vi "Download Record.vi"(0 "Instrument Handle In":i32, 1 "Start Time":dbl format="%^#_6g", 5 "Source":i32(ring) items=["Input Channel 1", "Input Channel 2", "Input Channel 3", "Input Channel 4", "Calc Channel 1", "Calc Channel 2", "Calc Channel 3", "Calc Channel 4", "Ref Channel 1", "Ref Channel 2", "Ref Channel 3", "Ref Channel 4"], 7 "Points":i32=1000, 9 "Transfer Type":i32(ring)=2 items=["s8", "s16", "s32", "f32", "f64"], 11 "error in":errorcluster, 12 "Stop Time":dbl format="%^#_6g") -> (3 "F64 Wave":dbl[](array[numeric]), 4 "Instrument Handle Out":i32, 6 "S8 Wave":i8[](array[numeric]), 8 "S16 Wave":i16[](array[numeric]), 10 "S32 Wave":i32[](array[numeric]), 14 "F32 Wave":sgl[](array[numeric]), 15 "error out":errorcluster)   [LabVIEW 2013, in "ZTScopeM.lvlib"]
doc: "Read the waveform in the source channel. The returned data format depends on the Transfer Type. Use \"Read Waveform Preamble\" to get the appropriate time and magnitude bases."
uses:
  ZTScopeM.lvlib
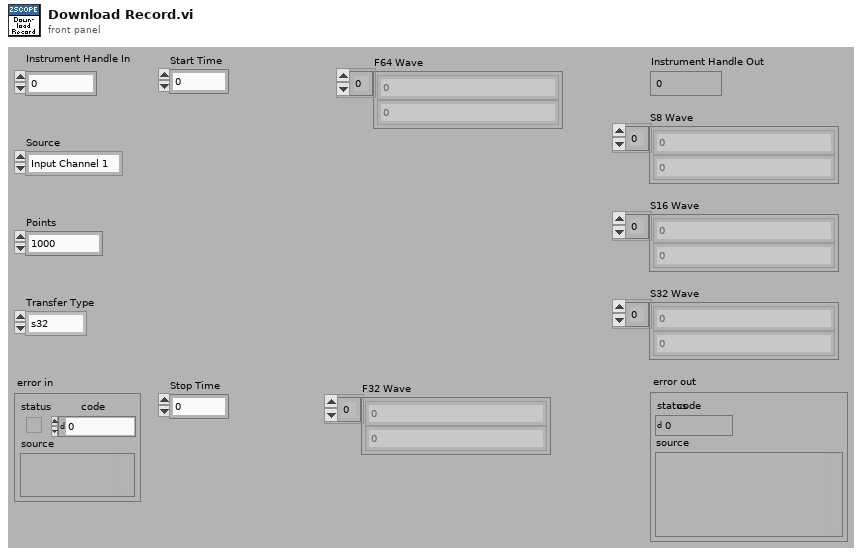
[diagram p1: front panel]
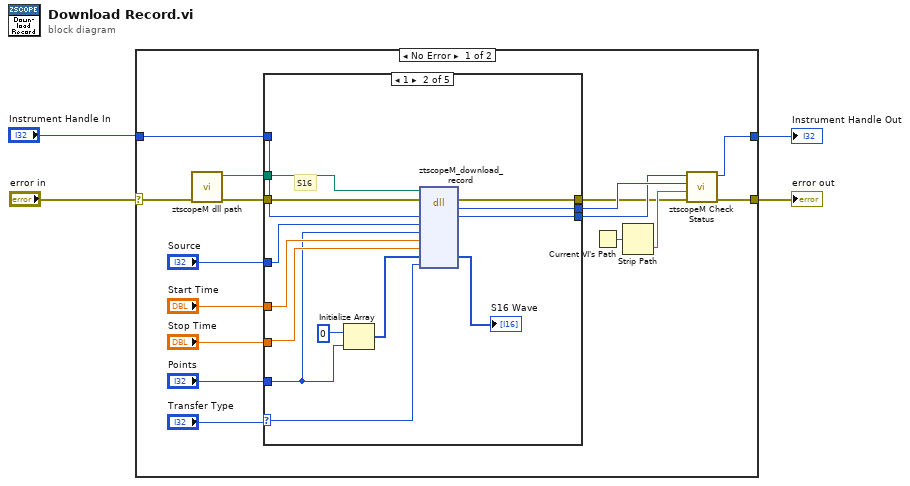
[diagram p0: block diagram]
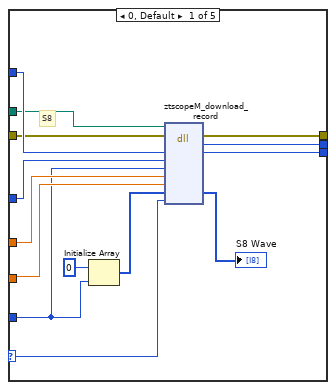
[diagram p2: hidden frame]
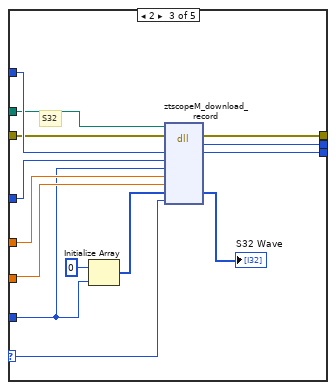
[diagram p3: hidden frame]
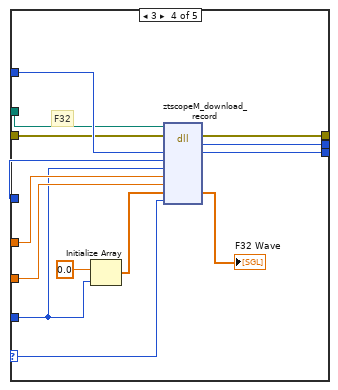
[diagram p4: hidden frame]
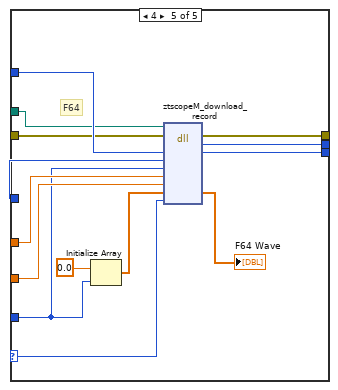
[diagram p5: hidden frame]
diagram:
  n1 = case shown="No Error" "error in" {
    selector: "error in" -> [w8 w92]
    tunnel: [w15 w92] -> w1
    tunnel: "Instrument Handle In" -> [w14 w91]
    tunnel: [w16 w91] -> w3
    frame No Error {
      n2 = call "ztscopeM dll path.vi"("error in (no error)"=w8) -> ("error out"=w6:errorcluster, "<instrument>.dll path"=w7:path)  [unwired: 9 in]
      n3 = case shown="1" "Transfer Type" {
        selector: "Transfer Type" -> [w25 w39 w53 w67 w81]
        tunnel: [w27 w41 w55 w75 w89] -> w18
        tunnel: [w26 w40 w54 w74 w88] -> w17
        tunnel: w14 -> [w28 w42 w56 w73 w87]
        tunnel: "Points" -> [w24 w38 w52 w66 w80]
        tunnel: "Source" -> [w29 w43 w57 w72 w86]
        tunnel: "Start Time" -> [w30 w44 w58 w69 w83]
        tunnel: "Stop Time" -> [w31 w45 w59 w68 w82]
        tunnel: w7 -> [w23 w37 w51 w65 w79]
        tunnel: w6 -> [w22 w36 w49 w64 w78]
        tunnel: [w21 w35 w50 w63 w77] -> w5
        frame 0, Default {
          # "S8"
          n4 = Initialize Array(i8 0, w24) -> (w33:i8[])
          n5 = dll-call lib="C:/Program Files (x86)/National Instruments/LabVIEW 2013/instr.lib/ztscopem/ztscopeM.dll" fn="ztscopeM_download_record"(path in=w23, error in=w22, "instrumentHandle"=w28, "source"=w29, "points"=w24, "startTime"=w30, "stopTime"=w31, "Waveform"=w33, "transferType"=w25) -> (error out=w21:errorcluster, w27:i32, "instrumentHandle"=w26:i32, "Waveform"=→"S8 Wave":i8[])  [unwired: 6 in, 1 out]
        }
        frame 1 {
          # "S16"
          n6 = Initialize Array(i16 0, w38) -> (w47:i16[])
          n7 = dll-call lib="C:/Program Files (x86)/National Instruments/LabVIEW 2013/instr.lib/ztscopem/ztscopeM.dll" fn="ztscopeM_download_record"(path in=w37, error in=w36, "instrumentHandle"=w42, "source"=w43, "points"=w38, "startTime"=w44, "stopTime"=w45, "Waveform"=w47, "transferType"=w39) -> (error out=w35:errorcluster, w41:i32, "instrumentHandle"=w40:i32, "Waveform"=→"S16 Wave":i16[])  [unwired: 6 in, 1 out]
        }
        frame 2 {
          # "S32"
          n8 = Initialize Array(0, w52) -> (w61:i32[])
          n9 = dll-call lib="C:/Program Files (x86)/National Instruments/LabVIEW 2013/instr.lib/ztscopem/ztscopeM.dll" fn="ztscopeM_download_record"(path in=w51, error in=w49, "instrumentHandle"=w56, "source"=w57, "points"=w52, "startTime"=w58, "stopTime"=w59, "Waveform"=w61, "transferType"=w53) -> (error out=w50:errorcluster, w55:i32, "instrumentHandle"=w54:i32, "Waveform"=→"S32 Wave":i32[])  [unwired: 6 in, 1 out]
        }
        frame 3 {
          # "F32"
          n10 = Initialize Array(sgl 0.0, w66) -> (w71:sgl[])
          n11 = dll-call lib="C:/Program Files (x86)/National Instruments/LabVIEW 2013/instr.lib/ztscopem/ztscopeM.dll" fn="ztscopeM_download_record"(path in=w65, error in=w64, "instrumentHandle"=w73, "source"=w72, "points"=w66, "startTime"=w69, "stopTime"=w68, "Waveform"=w71, "transferType"=w67) -> (error out=w63:errorcluster, w75:i32, "instrumentHandle"=w74:i32, "Waveform"=→"F32 Wave":sgl[])  [unwired: 6 in, 1 out]
        }
        frame 4 {
          # "F64"
          n12 = Initialize Array(0.0, w80) -> (w85:dbl[])
          n13 = dll-call lib="C:/Program Files (x86)/National Instruments/LabVIEW 2013/instr.lib/ztscopem/ztscopeM.dll" fn="ztscopeM_download_record"(path in=w79, error in=w78, "instrumentHandle"=w87, "source"=w86, "points"=w80, "startTime"=w83, "stopTime"=w82, "Waveform"=w85, "transferType"=w81) -> (error out=w77:errorcluster, w89:i32, "instrumentHandle"=w88:i32, "Waveform"=→"F64 Wave":dbl[])  [unwired: 6 in, 1 out]
        }
      }
      n14 = Current VI's Path() -> (path=w20:path)
      n15 = Strip Path(path=w20) -> (name=w19:string)  [unwired: 1 out]
      n16 = call "ztscopeM Check Status.vi"("error in"=w5, "name of VI"=w19, "status (return code)"=w18, "instrument handle in"=w17) -> ("error out"=w15:errorcluster, "instrument handle out"=w16:i32)  [unwired: 2 in]
    }
    frame Error {
    }
  }
  "Instrument Handle Out" <- w3
  "error out" <- w1
